vi "ChangeClfnErrorCheckingLevel.vi"() -> ()   [LabVIEW 2016]
uses:
  <vilib>/Utility/traverseref.llb/TRef TravTarget.ctl
  <vilib>/Utility/traverseref.llb/VI Scripting - Traverse.lvlib
panel:
  in  "Folder Path":path
  out "All Files in Dir":path[](array[path])
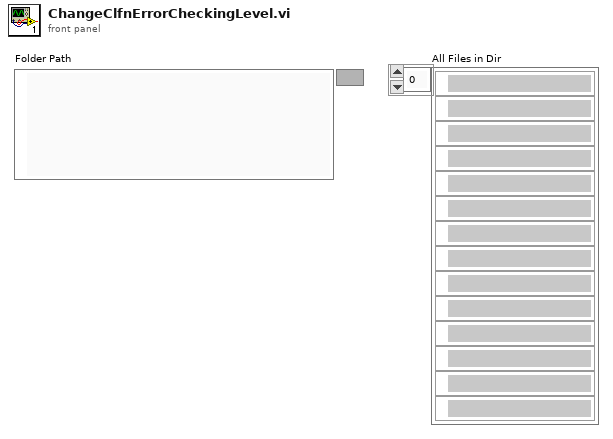
[diagram p1: front panel]
types:
  T1 = typedef "TRef TravTarget.ctl" = enum16{"FP", "BD", "Other"}
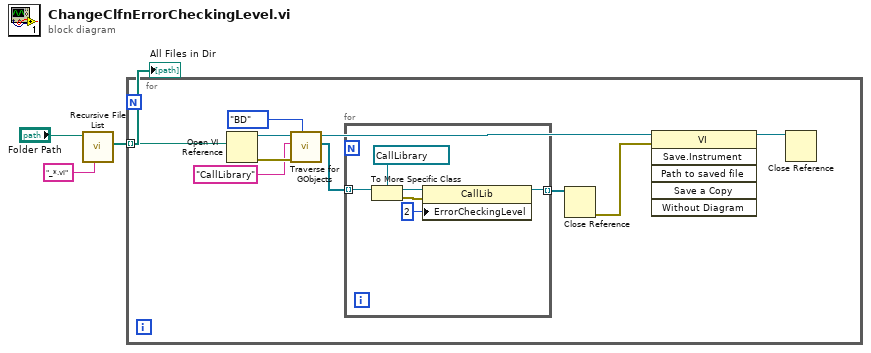
[diagram p0: block diagram]
diagram:
  n1 = call <vilib>:"Recursive File List.vi"("pattern"="_*.vi", "Folder Path"="Folder Path") -> ("All Files in Dir"=w1:path[])  [unwired: 5 in, 4 out]
  "All Files in Dir" <- w1
  n2 = for {
    tunnel: w1 -> [w13] mode=indexing
    n3 = Open VI Reference(vi path=w13) -> (vi reference=w11:refnum<vi>, error out=w12:errorcluster)  [unwired: 5 in]
    n4 = call <vilib>:"Traverse for GObjects.vi"("Traverse Target"=TRef_TravTarget."BD", "error in (no error)"=w12, "Class Name"="CallLibrary", "VI Refnum"=w11) -> ("References"=w8:refnum<vi>[], "dup VI Refnum"=w6:refnum<vi>)  [unwired: 4 in, 2 out]
    n5 = for {
      tunnel: w8 -> [w19] mode=indexing
      tunnel: [w14] -> w7 mode=indexing
      n6 = To More Specific Class(target class=refnum<vi> refnum ("Other Refnum"), reference=w19) -> (specific class reference=w17:refnum<vi>, error out=w16:errorcluster)  [unwired: 1 in]
      n7 = property class="CallLib"(reference=w17, error in=w16, "ErrorCheckingLevel"=u32 2 ("Error Checking Level")) -> (reference out=w14:refnum<vi>)  [unwired: 1 out]
    }
    n8 = Close Reference(reference=w7) -> (error out=w5:errorcluster)  [unwired: 1 in]
    n9 = invoke class="VI" method="Save.Instrument"(reference=w6, error in=w5) -> (reference out=w4:refnum<vi>)  [unwired: 4 in, 5 out]
    n10 = Close Reference(reference=w4) -> ()  [unwired: 1 in, 1 out]
  }
